vi "write electrical data.vi"(8 "error in (no error)":errorcluster, 10 "Electrical Data 2":T1, 11 "Metadata":string[][](array[string])) -> (0 "error out":errorcluster)   [LabVIEW 2013]
uses:
  Controls/electrical.ctl
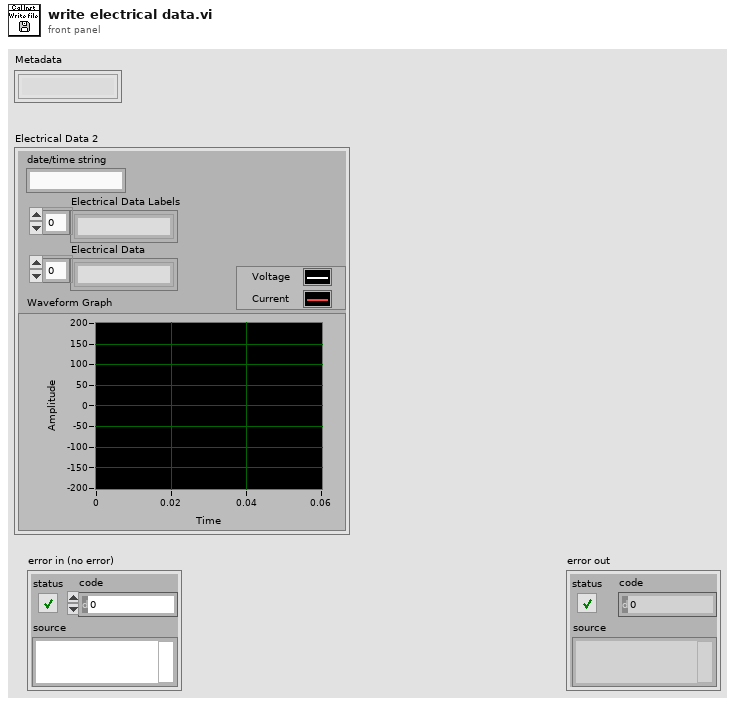
[diagram p1: front panel]
types:
  T1 = typedef "electrical.ctl" = cluster{"date/time string":string, "Electrical Data Labels":string[], "Electrical Data":string[], "Waveform Graph":waveform(dbl)[]}
  T2 = enum16{"open", "open or create", "create or replace", "create", "open (read-only)"}
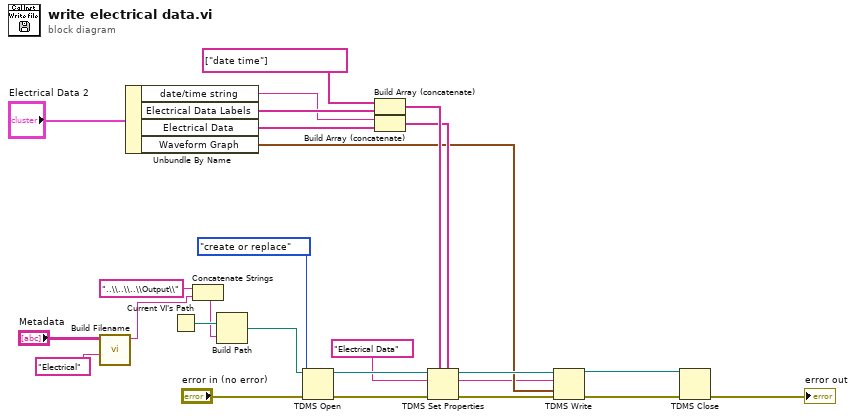
[diagram p0: block diagram]
diagram:
  n1 = call "Build Filename.vi"("Measurment Type"="Electrical", "Metadata In"="Metadata") -> ("String"=w1:string)  [unwired: 9 in]
  n2 = Unbundle By Name("Electrical Data 2") -> ("date/time string"=w17:string, "Electrical Data Labels"=w19:string[], "Electrical Data"=w16:string[], "Waveform Graph"=w13:waveform(dbl)[])
  n3 = Current VI's Path() -> (path=w10:path)
  n4 = Concatenate Strings("..\\..\\..\\Output\\" ("string"), w1) -> (w2:string)
  n5 = Build Path(base path=w10, name or relative path=w2) -> (appended path=w9:path)
  n6 = TDMS Open(8:"error in (no error)", 10:T2."create or replace" ("operation (0:open)"), 11:w9) -> (0:w24:errorcluster, 3:w25:refnum<k34>)  [unwired: 4 in]
  n7 = Build Array (concatenate)(string[] ["date time"] ("element"), w19) -> (w15:string[])
  n8 = Build Array (concatenate)(w17, w16) -> (w14:string[])
  n9 = TDMS Set Properties(5:w14, 7:w15, 8:w24, 10:"Electrical Data" ("group name"), 11:w25) -> (0:w22:errorcluster, 2:w6:string, 3:w23:refnum<k34>)  [unwired: 1 in, 1 out]
  n10 = TDMS Write(0:w23, 5:w6, 9:w13, 11:w22) -> (4:w21:refnum<k34>, 15:w20:errorcluster)  [unwired: 2 in, 2 out]
  n11 = TDMS Close(8:w20, 11:w21) -> (0:→"error out":errorcluster)  [unwired: 1 out]
